vi "Search JSON arr.vi"(8 "error in":errorcluster, 9 "Search Terms":string[](array[string])=["id"], 10 "Name of arr":string, 11 "Response body":string) -> (0 "error out":errorcluster, 3 "Respsonse":string[](array[string]))   [LabVIEW 2024, in "GUI.lvlib" / "Functions.lvlib"]
uses:
  Functions.lvlib
  <vilib>/addons/JSON API/JSON Value/Set from JSON string.vi
  <vilib>/addons/JSON API/JSON Value/Get Array by name.vi
  <vilib>/addons/JSON API/JSON Scalar/Get as Text.vi
  <vilib>/addons/JSON API/JSON Value/JSON Value.lvclass
  <vilib>/addons/JSON API/Get Polymorphic/JSON GetSet.lvlib
  <vilib>/addons/JSON API/JSON Scalar/JSON Scalar.lvclass
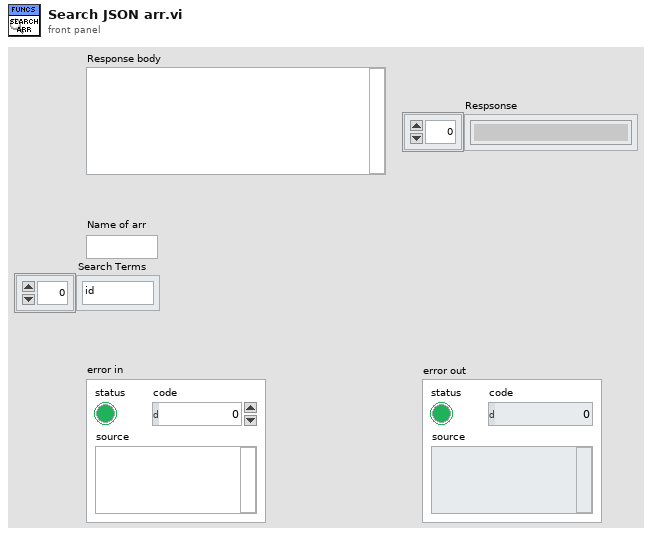
[diagram p1: front panel]
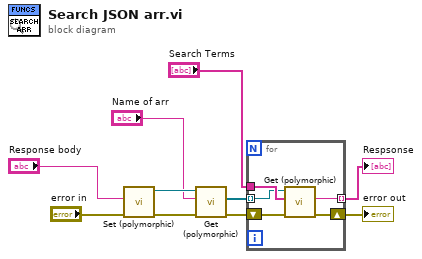
[diagram p0: block diagram]
diagram:
  n1 = call-poly <vilib>:"Set (polymorphic).vi"("error in (no error)"="error in", "JSON stream"="Response body") -> ("error out"=w5:errorcluster, "JSON Value out"=w6:refnum<class "JSON Value.lvclass">)  [unwired: 7 in, 1 out]
  n2 = call-poly <vilib>:"Get (polymorphic).vi"("error in (no error)"=w5, "name"="Name of arr", "JSON Value In"=w6) -> ("error out"=w4:errorcluster, "Array"=w2:refnum<class "JSON Value.lvclass">[])  [unwired: 5 in, 2 out]
  n3 = for {
    tunnel: [w15] -> w9 mode=indexing
    tunnel: "Search Terms" -> [w12]
    shift-right: [w14] -> w8
    shift-left: w4 -> [w13]
    tunnel: w2 -> [w11] mode=indexing
    n4 = call-poly <vilib>:"Get (polymorphic).vi"("error in (no error)"=w13, "Name Array"=w12, "JSON Scalar in"=w11) -> ("error out"=w14:errorcluster, "LabVIEW Text"=w15:string)  [unwired: 6 in, 1 out]
  }
  "error out" <- w8
  "Respsonse" <- w9
